vi "Write Scan Channels.vi"(8 "error in (no error)":errorcluster, 10 "Scan Channels":i32[](array[numeric]), 11 "LR-700 Driver in":refnum<class "LR-700 Driver.lvclass">) -> (0 "error out":errorcluster, 3 "LR-700 Driver out":refnum<class "LR-700 Driver.lvclass">)   [LabVIEW 2015, in "LR-700 Driver.lvclass"]
uses:
  LR-700 Driver.lvclass
  LR-700 Driver.lvclass/LR-700 Driver.ctl
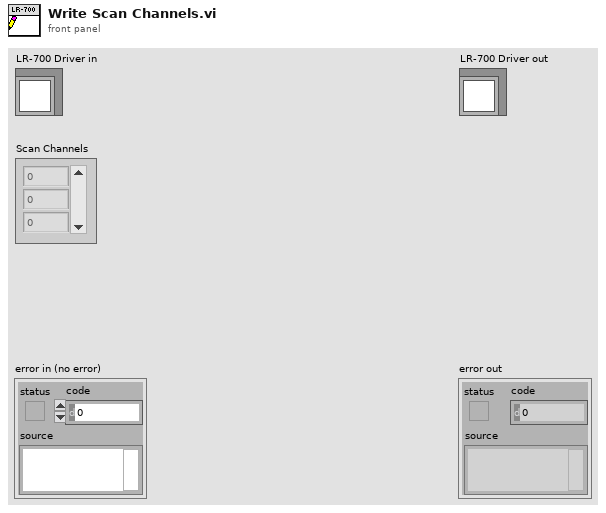
[diagram p1: front panel]
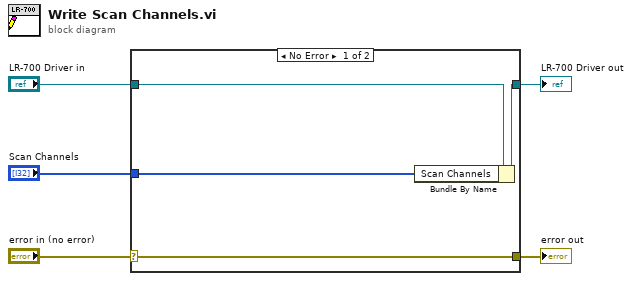
[diagram p0: block diagram]
diagram:
  n1 = case shown="No Error" "error in (no error)" {
    selector: "error in (no error)" -> [w9 w10]
    tunnel: [w9 w10] -> w4
    tunnel: [w7 w11] -> w2
    tunnel: "LR-700 Driver in" -> [w8 w11]
    tunnel: "Scan Channels" -> [w6 _]
    frame No Error {
      n2 = Bundle By Name(cluster=w8, "Scan Channels"=w6) -> (w7:refnum<class "LR-700 Driver.lvclass">)
    }
    frame Error {
    }
  }
  "error out" <- w4
  "LR-700 Driver out" <- w2
